vi "L0ManualControl.vi"() -> ()   [LabVIEW 2012]
panel:
  out "Delay Index":u16(ring) items=["0", "0.25ns", "0.5ns", "0.75ns", "1ns", "1.25ns", "1.5ns", "1.75ns", "2ns", "2.25ns", "2.5ns", "2.75ns", "3ns", "3.25ns", "3.5ns", "3.75ns", "4ns", "4.25ns", "4.5ns", "4.75ns", "5ns", "5.25ns", "5.5ns", "5.75ns", "2ns_b", "2.25ns_b", "2.5ns_b", "2.75ns_b", "3ns_b", "3.25ns_b", "3.5ns_b", "3.75ns_b", ""]
  out "Ib_Clipping":i32
  out "Clipping":i32
  out "Attenuation":i32
  out "Channel":i32
  in  "stop":bool
  in  "Ib Clipping Select":i32(slide) scale=1.0..32.0
  in  "Clipping Select":i32(slide) scale=1.0..3.0
  in  "Attenuation Select":i32(slide) scale=0.0..12.0
  in  "Delay Select":i32(slide) scale=0.0..31.0
  in  "Channel Select":i32(slide) scale=0.0..6.0
  out "VISA resource name out":refnum<visa-resource-name>="Oscilloscope"
  out "error 2 out":errorcluster
  in  "error in 1":errorcluster
  in  "Osc":refnum<visa-resource-name>="Oscilloscope"
  in  "Generator":refnum<visa-resource-name>="generadorpulsos"
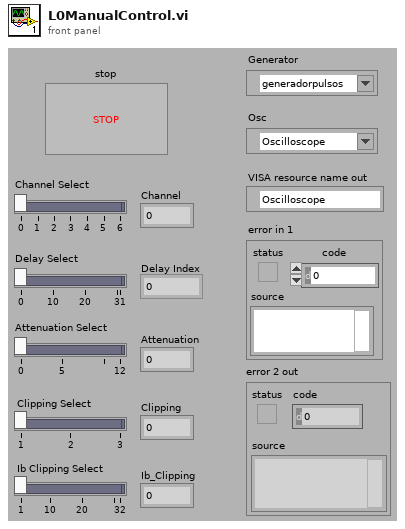
[diagram p1: front panel]
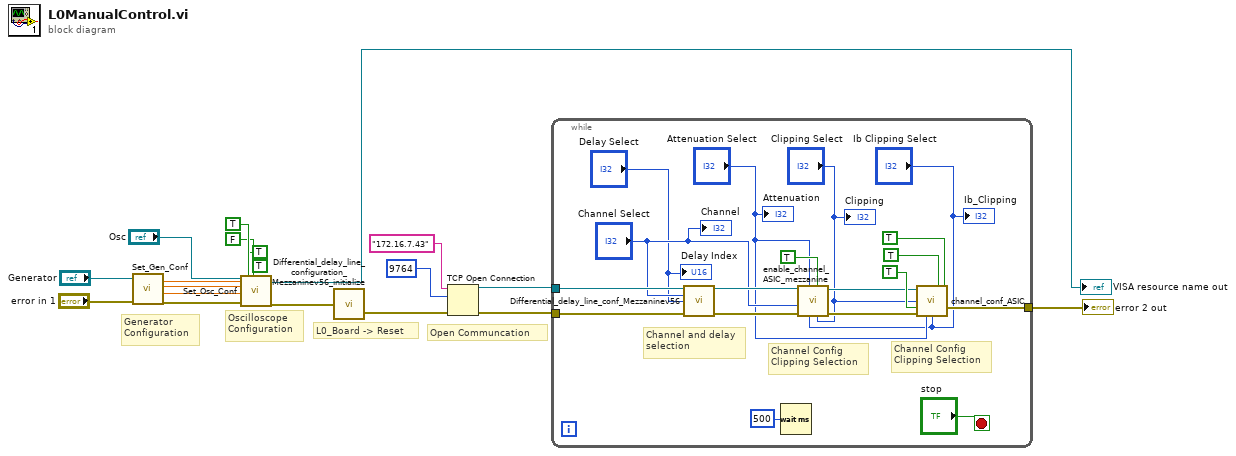
[diagram p0: block diagram]
diagram:
  # "Open Communcation"
  # "Oscilloscope\nConfiguration"
  # "Generator \nConfiguration"
  # "L0_Board -> Reset"
  n1 = call "Set_Gen_Conf.vi"("AWG VISA"="Generator", "error in (no error)"="error in 1") -> ("Amplitude 1 OUT"=w12:dbl, "Pulse Width in seconds 1 OUT"=w5:dbl, "Trigger Level 1"=w6:dbl, "error out"=w11:errorcluster)  [unwired: 10 in, 4 out]
  n2 = call "Set_Osc_Conf.vi"("VISA resource name"="Osc", "Amplitude IN"=w12, "Trigger Level IN"=w6, "Pulse Width in seconds IN"=w5, "error in (no error)"=w11, "Channel 1"=TRUE, "Channel 3"=TRUE, "Channel 2"=FALSE, "Channel 4"=TRUE) -> ("VISA resource name out"=→"VISA resource name out":refnum<visa-resource-name>, "error out"=w10:errorcluster)  [unwired: 9 in]
  n3 = call "Differential_delay_line_configuration_Mezzaninev56_initialize.vi"("error in (no error)"=w10) -> ("error out 2"=w7:errorcluster)  [unwired: 1 in]
  n4 = TCP Open Connection(address="172.16.7.43", remote port or service name=u16 9764, error in (no error)=w7) -> (connection ID=w1:refnum<k5>, error out=w2:errorcluster)  [unwired: 2 in]
  n5 = while {
    tunnel: [w32] -> w4
    tunnel: w2 -> [w31]
    tunnel: w1 -> [w29]
    stop <- "stop" stop-if-true
    # "Channel Config\nClipping Selection"
    # "Channel Config\nClipping Selection"
    # "Channel and delay\nselection"
    n6 = call "Differential_delay_line_conf_Mezzaninev56.vi"("connection ID"=w29, "channel"="Channel Select", "Delay value"="Delay Select", "error in (no error)"=w31) -> ("connection ID out"=w28:refnum<k5>, "error out 2"=w30:errorcluster)  [unwired: 4 in, 6 out]
    n7 = Wait (ms)(milliseconds to wait=500) -> ()  [unwired: 1 out]
    n8 = call "enable_channel_ASIC_mezzanine.vi"("Clip_sel_b"="Clipping Select", "maj/sum"=TRUE ("Att_en_b"), "Ib_clipVb"="Ib Clipping Select", "Att gain"="Attenuation Select", "error in"=w30, "Channel"="Channel Select", "connection ID"=w28) -> ("error out"=w36:errorcluster, "connection ID out"=w35:refnum<k5>)  [unwired: 2 in, 1 out]
    n9 = call "channel_conf_ASIC.vi"("connection ID"=w35, "Clip_sel_b"="Clipping Select", "CompBuf_en_b"=TRUE, "error out"=w36, "Att gain"="Attenuation Select", "Ib_ClipVb"="Ib Clipping Select", "Clip_en_b"=TRUE, "Att_en_b"=TRUE) -> ("error out 2"=w32:errorcluster)  [unwired: 3 in, 4 out]
    "Channel" <- "Channel Select"
    "Delay Index" <- "Delay Select"
    "Attenuation" <- "Attenuation Select"
    "Clipping" <- "Clipping Select"
    "Ib_Clipping" <- "Ib Clipping Select"
  }
  "error 2 out" <- w4
